vi "Build String Request.vi"(9 "Time Stamp In":timestamp, 10 "String Value In":string, 11 "Node ID In":string) -> (3 "Request Out":T3 {"node status" items=["Good"=0, "Uncertain"=1073741824, "Uncertain_InitialValue"=1083310080, "Uncertain_LastUsableValue"=1083179008, "Uncertain_SensorNotAccurate"=1083375616, "Uncertain_EngineeringUnitsExceeded"=1083441152, "Bad"=2147483648, "Bad_NoCommunication"=2150694912, "Bad_NotReadable"=2151284736, "Bad_NotWritable"=2151350272, "Bad_OutOfRange"=2151415808, "Bad_WaitingForInitialData"=2150760448]})   [LabVIEW 2024]
uses:
  <vilib>/OPCUA/controls/Write Status.ctl
  <vilib>/OPCUA/controls/NodeId.ctl
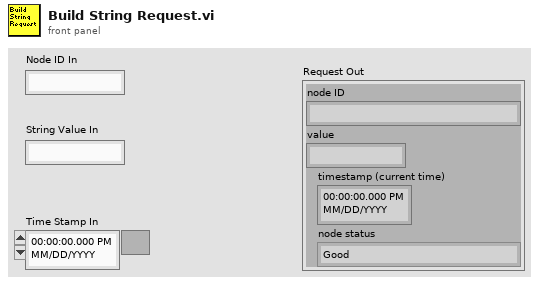
[diagram p1: front panel]
types:
  T1 = typedef "NodeId.ctl" = string
  T2 = typedef "Write Status.ctl" = u32
  T3 = cluster{"node ID":T1, "value":string, "timestamp (current time)":timestamp, "node status":T2}
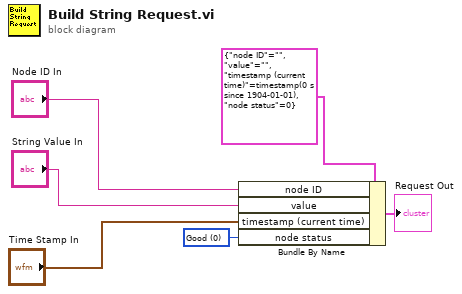
[diagram p0: block diagram]
diagram:
  w2 = T2 0 items=["Good"=0, "Uncertain"=1073741824, "Uncertain_InitialValue"=1083310080, "Uncertain_LastUsableValue"=1083179008, "Uncertain_SensorNotAccurate"=1083375616, "Uncertain_EngineeringUnitsExceeded"=1083441152, "Bad"=2147483648, "Bad_NoCommunication"=2150694912, "Bad_NotReadable"=2151284736, "Bad_NotWritable"=2151350272, "Bad_OutOfRange"=2151415808, "Bad_WaitingForInitialData"=2150760448] ("node status")
  n1 = Bundle By Name(cluster=T3 {"node ID"="", "value"="", "timestamp (current time)"=timestamp(0 s since 1904-01-01), "node status"=0} ("request"), "node ID"="Node ID In", "value"="String Value In", "timestamp (current time)"="Time Stamp In", "node status"=w2) -> (→"Request Out":T3)
